vi "SensorRefNums.vi"() -> (0 "Sensors":T1={"ElevatorBottom"={"DeviceStatus"={"status"=FALSE, "code"=0, "source"=""}, "Device Number"=0, "Handle"=0, "Library Path"=path ""}, "ElevatorTop"={"DeviceStatus"={"status"=FALSE, "code"=0, "source"=""}, "Device Number"=0, "Handle"=0, "Library Path"=path ""}, "ControlPanelColor"={"DevStatus"={"status"=FALSE, "code"=0, "source"=""}, "Device Address"=0, "Handle"=0, "I2C Bus"=enum."Invalid"}} {"ControlPanelColor"."Device Address" format="%.0x"; "ElevatorBottom"."Handle" format="%x"; "ElevatorTop"."Handle" format="%x"})   [LabVIEW 2019]
uses:
  TypeDefs/RobotComponents/SensorRefNums.ctl
  <vilib>/Playing With Fusion Inc/Playing With Fusion Lib for FRC/PWF_ToF_LabVIEW/Public/TypeDefs/PwF_ToF_DevRef.ctl
  <vilib>/Playing With Fusion Inc/Playing With Fusion Lib for FRC/PWF_TMD37003_LabVIEW/Public/TypeDefs/PwF_TMD37003_DevRef.ctl
  <vilib>/Rock Robotics/SystemInterfaces/i2clib/i2c_bus.ctl
  <vilib>/Playing With Fusion Inc/Playing With Fusion Lib for FRC/PWF_ToF_LabVIEW/PwF_ToF.lvlib
  <vilib>/Playing With Fusion Inc/Playing With Fusion Lib for FRC/PWF_TMD37003_LabVIEW/PwF_TMD37003.lvlib
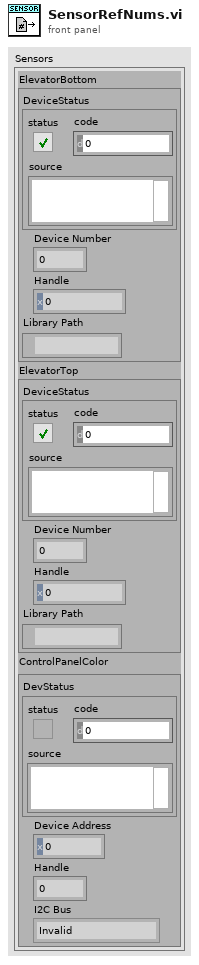
[diagram p1: front panel]
types:
  T1 = typedef "SensorRefNums.ctl" = cluster{"ElevatorBottom":T2, "ElevatorTop":T2, "ControlPanelColor":T3}
  T2 = typedef "PlayingWithFusionLib.lvlib/PwF_ToF.lvlib/PwF_ToF_DevRef.ctl" = cluster{"DeviceStatus":errorcluster, "Device Number":u8, "Handle":u64, "Library Path":path}
  T3 = typedef "PlayingWithFusionLib.lvlib/PwF_TMD37003.lvlib/PwF_TMD37003_DevRef.ctl" = cluster{"DevStatus":errorcluster, "Device Address":u8, "Handle":i32, "I2C Bus":T4}
  T4 = typedef "i2c_bus.ctl" = enum16{"I2C On-Board", "I2C MXP", "Invalid"}
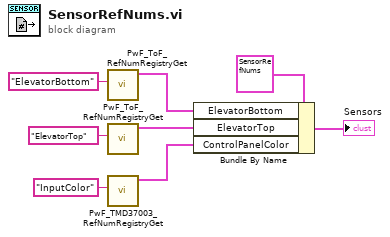
[diagram p0: block diagram]
diagram:
  n1 = call <vilib>:"PwF_ToF_RefNumRegistryGet.vi"("refnum name"="ElevatorBottom") -> ("PwFToFDevRefOut"=w8:T2)  [unwired: 9 in, 1 out]
  n2 = call <vilib>:"PwF_ToF_RefNumRegistryGet.vi"("refnum name"="ElevatorTop") -> ("PwFToFDevRefOut"=w7:T2)  [unwired: 9 in, 1 out]
  n3 = call <vilib>:"PwF_TMD37003_RefNumRegistryGet.vi"("refnum name"="InputColor") -> ("PwFTMD37003DevRefOut"=w2:T3)  [unwired: 9 in, 1 out]
  n4 = Bundle By Name(cluster=T1 {"ElevatorBottom"={"DeviceStatus"={"status"=FALSE, "code"=0, "source"=""}, "Device Number"=0, "Handle"=0, "Library Path"=path ""}, "ElevatorTop"={"DeviceStatus"={"status"=FALSE, "code"=0, "source"=""}, "Device Number"=0, "Handle"=0, "Library Path"=path ""}, "ControlPanelColor"={"DevStatus"={"status"=FALSE, "code"=0, "source"=""}, "Device Address"=0, "Handle"=0, "I2C Bus"=enum."Invalid"}} ("output cluster"), "ElevatorBottom"=w8, "ElevatorTop"=w7, "ControlPanelColor"=w2) -> (→"Sensors":T1)
